vi "New Assert Message.vi"(8 "error in (no error)":errorcluster, 10 "Assert Message":T1, 11 "Single Assert Display in":refnum<class "Single Assert Display.lvclass">) -> (0 "error out":errorcluster, 3 "Single Assert Display out":refnum<class "Single Assert Display.lvclass">)   [LabVIEW 2016, in "Assert API Components.lvlib" / "Assert Display.lvlib" / "Single Assert Display.lvlib" / "Single Assert Display.lvclass"]
uses:
  Single Assert Display.lvclass
  Assert API Components/Message Data.ctl
  Assert API Components/VI References.ctl
  Single Assert Display.lvclass/Single Assert Display.ctl
  Assert API Components/Assert API Components.lvlib
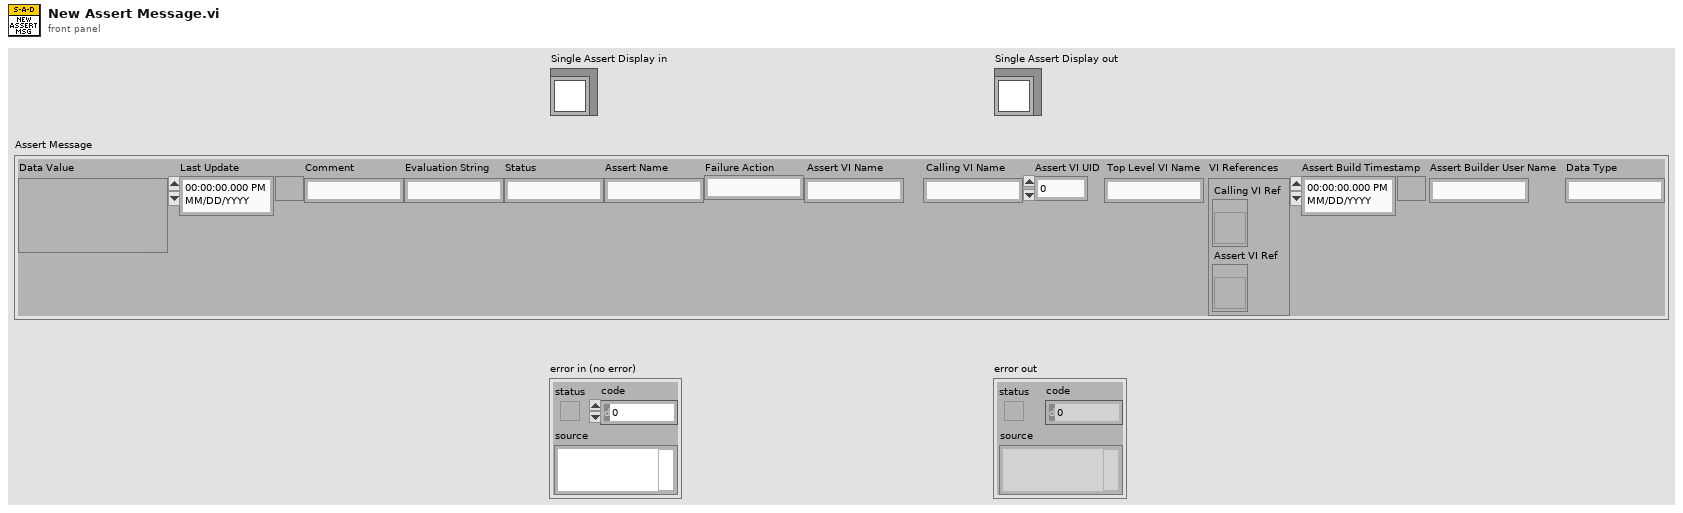
[diagram p1: front panel]
types:
  T1 = typedef "Assert API Components.lvlib/Message Data.ctl" = cluster{"Data Value":variant, "Last Update":timestamp, "Comment":string, "Evaluation String":string, "Status":string, "Assert Name":string, "Failure Action":string, "Assert VI Name":string, "Calling VI Name":string, "Assert VI UID":i32, "Top Level VI Name":string, "VI References":T2, "Assert Build Timestamp":timestamp, "Assert Builder User Name":string, "Data Type":string}
  T2 = typedef "Assert API Components.lvlib/VI References.ctl" = cluster{"Calling VI Ref":refnum<vi>, "Assert VI Ref":refnum<vi>}
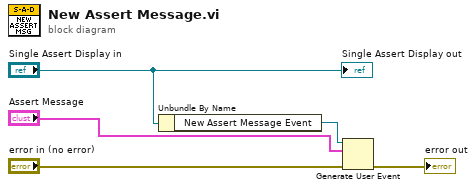
[diagram p0: block diagram]
diagram:
  n1 = Unbundle By Name("Single Assert Display in") -> ("New Assert Message Event"=w2:refnum<user-event>)
  n2 = Generate User Event(user event=w2, event data cluster="Assert Message", error in="error in (no error)") -> (error out=→"error out":errorcluster)  [unwired: 1 in, 1 out]
  "Single Assert Display out" <- "Single Assert Display in"
